vi "CRYSave Operator Window Configure.vi"(8 "error in":errorcluster, 11 "Save Mode":string) -> (0 "error out":errorcluster)   [LabVIEW 2013]
uses:
  SubVI/CRYMisc vis settings global.vi
  CRYMainGlobal.vi
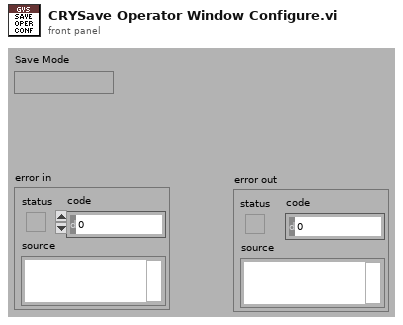
[diagram p1: front panel]
types:
  T1 = enum16{"Left Button", "Center Button", "Right Button", "Window Close"}
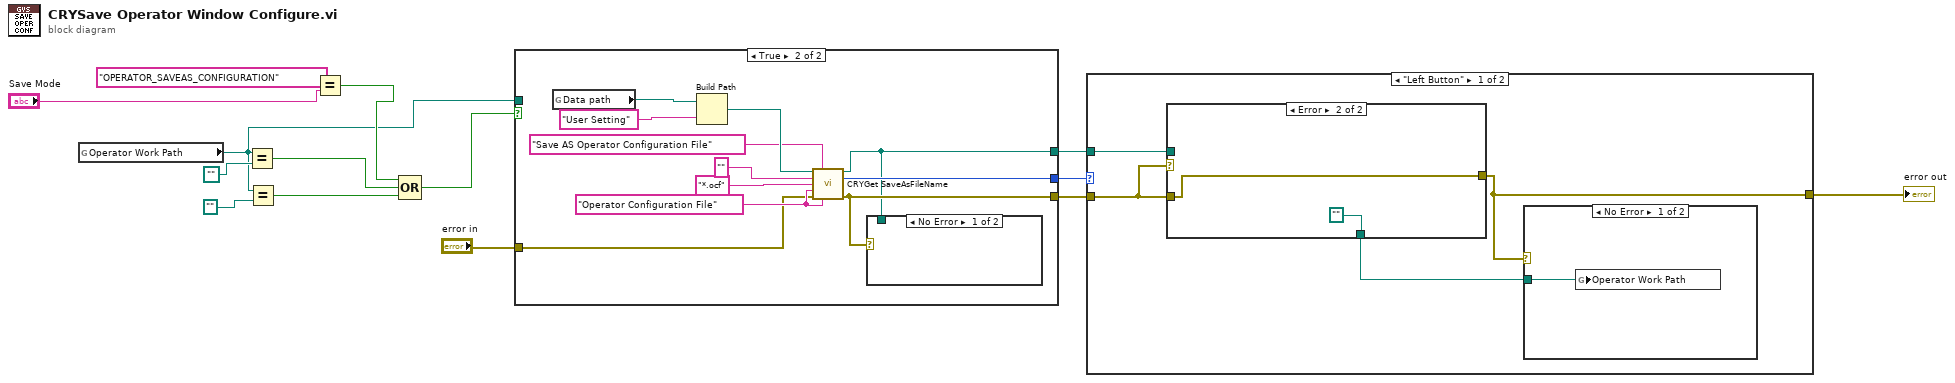
[diagram p0: block diagram]
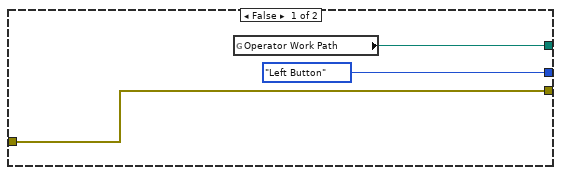
[diagram p2: hidden frame]
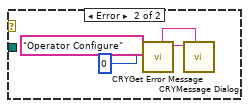
[diagram p4: hidden frame]
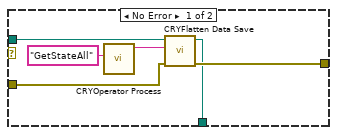
[diagram p5: hidden frame]
diagram:
  n1 = global read "CRYMisc vis settings global.vi" "Operator Work Path"() -> (w1:path)
  n2 = Equal?(x=w1, y=path "") -> (x = y?=w7:bool)
  n3 = Equal?(x=w1, y=path "") -> (x = y?=w6:bool)
  n4 = Equal?(x="OPERATOR_SAVEAS_CONFIGURATION" ("Save Mode"), y="Save Mode") -> (x = y?=w5:bool)
  n5 = Compound Arithmetic op=OR(w5, w7, w6) -> (w4:bool)
  n6 = case shown="True" w4 {
    tunnel: [T1."Left Button" ("Which Button?") w23] -> w14
    tunnel: [w15 w20] -> w13
    tunnel: [w17 w21] -> w12
    tunnel: "error in" -> [w17 w22]
    tunnel: w1 -> [_ _]
    frame False {
      n7 = global read "CRYMisc vis settings global.vi" "Operator Work Path"() -> (w15:path)
    }
    frame True {
      w25 = "Operator Configuration File" ("pattern label")
      n8 = global read "CRYMainGlobal.vi" "Data path"() -> (w19:path)
      n9 = Build Path(base path=w19, name or relative path="User Setting") -> (appended path=w27:path)
      n10 = call "CRYGet SaveAsFileName.vi"("Start path"=w27, "TitleName"="Save AS Operator Configuration File" ("prompt"), "default name"="", "pattern (all files)"="*.ocf", "pattern label"=w25, "error in"=w22, "Category Name"=w25) -> ("Path"=w20:path, "Which Button?"=w23:T1, "error out"=w21:errorcluster)  [unwired: 2 in, 4 out]
      n11 = case shown="No Error" w21 {
        tunnel: w20 -> [_ _]
        frame No Error {
        }
        frame Error {
        }
      }
    }
  }
  n12 = case shown="\"Left Button\"" w14 {
    tunnel: w13 -> [w32 _]
    tunnel: w12 -> [w31 w46]
    tunnel: [w30 w46] -> w2
    frame "Left Button" {
      n13 = case shown="Error" w31 {
        tunnel: w31 -> [w43 w45]
        tunnel: [w42 w45] -> w30
        tunnel: w32 -> [w41 _]
        tunnel: [w38 path ""] -> w29
        frame No Error {
          n14 = call "CRYOperator Process.vi"("sAction"="GetStateAll") -> ("Data String"=w39:string)  [unwired: 10 in]
          n15 = call "CRYFlatten Data Save.vi"("error in"=w43, "Any Flatten Data"=w39, "Path In"=w41) -> ("error out"=w42:errorcluster, "Path Out"=w38:path)  [unwired: 5 in]
        }
        frame Error {
        }
      }
      n16 = case shown="No Error" w30 {
        tunnel: w29 -> [w33 _]
        frame No Error {
          n17 = global write "CRYMisc vis settings global.vi" "Operator Work Path"(w33) -> ()
        }
        frame Error {
          n18 = call "CRYGet Error Message.vi"("Error No"=0, "Kind"="Operator Configure") -> ("Message"=w37:string, "Window Title"=w36:string)  [unwired: 4 in, 4 out]
          n19 = call "CRYMessage Dialog.vi"("Window Title"=w36, "Message Content"=w37) -> ()  [unwired: 8 in, 2 out]
        }
      }
    }
    frame "Center Button", Default {
    }
  }
  "error out" <- w2
